vi "FPGA (Test Encoders).vi"() -> ()   [LabVIEW 2017]
uses:
  <vilib>/Platform/TimedLoop/XDataNode/timing_clust.ctl
  <vilib>/Platform/TimedLoop/XDataNode/nitl_modes.ctl
  <vilib>/Platform/TimedLoop/XDataNode/wakeup.ctl
  <vilib>/rvi/Emulation/niFpgaSctlEmulationGetInTimedLoop.vi
  <vilib>/rvi/Emulation/niFpgaEmulationReportErrorSimple.vi
  <vilib>/rvi/Emulation/niFpgaGetClockAttributes.vi
  <vilib>/rvi/Emulation/niFpgaCriticalErrorInLSC.vi
  <vilib>/rvi/Emulation/niFpgaEmulationIsFPGAContextNoSignature.vi
  <vilib>/rvi/DataTransferAndStorage/Container/Common/niFpgaContainerGetUniqueNameForEmu.vi
  <vilib>/rvi/Memory/Memory_Emulation/niFpgaMemoryEmulationCacheClearOnFirstRun.vi
  <vilib>/rvi/Memory/Memory_Emulation/nirvimemoryEmulationManagerCache_MakeExclusive.vi
  <vilib>/rvi/Memory/Memory_Emulation/niFpgaMemoryEmulationValidateCache.vi
  <vilib>/rvi/Memory/Memory_Emulation/nirvimemoryEmulationManagerCache_InsertValue.vi
  <vilib>/Utility/error.llb/Clear Errors.vi
  <vilib>/rvi/Memory/Memory_Emulation/nirvimemoryEmulationManagerCache_ReleaseExclusive.vi
  <vilib>/rvi/Memory/Memory_Emulation/nirvimemoryEmulationManagerCache_GetValue.vi
  <vilib>/rvi/Memory/Memory_Emulation/nirvimemoryEmulationManagerCache_SetValue.vi
  <vilib>/rvi/Emulation/niFpgaProcessEmulError.vi
  <vilib>/rvi/eio/common/nirviEmuTemplateMethod_errors.vi
  <vilib>/Platform/TimedLoop/XDataNode/XDataNode.xnode
  <vilib>/rvi/DataTransferAndStorage/Container/XNode/niFpgaContainer.xnode
  <vilib>/rvi/DataTransferAndStorage/Register/Emulation/niFpgaRegisterEmulation.vi
  <vilib>/eio/EIONode/EIONode.xnode
  <vilib>/Platform/TimedLoop/XDataNode/XDNodeRunTimeDep.lvlib
panel:
  out "dENC2_POS":fxp<+/-,54,31>
  out "dENC1_POS":fxp<+/-,54,31>
  out "ENC_2_loop_count":i32
  out "ENC_1_loop_count":i32
  out "ENC2_ticks":i32
  out "ENC1_ticks":i32
  out "ENC2_POS":fxp<+/-,64,27>
  out "ENC1_POS":fxp<+/-,64,29>
  in  "ENC2_DEBOUNCE_CYCLES":u16=5
  in  "LINK2_ENC_CNTS 2":i32
  in  "LINK2_UPDATE_ENC 2":bool
  out "Link 2 Counts 2":i32
  out "Link 1 Counts":i32
  in  "ENC_DEBOUNCE_CYCLES":u16=5
  in  "LINK1_ENC_CNTS":i32
  in  "LINK1_UPDATE_ENC":bool
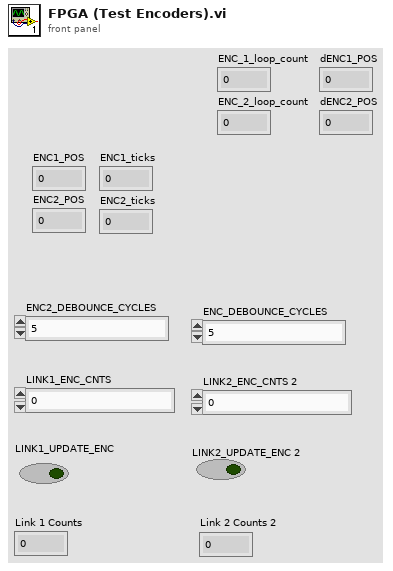
[diagram p1: front panel]
types:
  T1 = typedef "XDNodeRunTimeDep.lvlib/timing_clust.ctl" = cluster{"Expected End [f-1]":u64, "Actual End [f-1]":u64, "Finished Late? [f-1]":bool, "Expected End [i-1]":u64, "Actual End [i-1]":u64, "Finished Late? [i-1]":bool, "Expected Start [i]":u64, "Actual Start [i]":u64, "Expected Start [f]":u64, "Actual Start [f]":u64, "Source Name":string, "Structure Name":string, "Period":i64, "Deadline":i64, "Offset":i64, "Start":i64, "Priority":i32, "Timeout":i32, "Mode":T2, "Wakeup Reason":T3, "Error":errorcluster, "Source Type":string, "Secondary Source Type":string, "Global End Time":u64, "Global Start Time":u64, "Frame Duration":u64, "Iteration Duration":u64, "Assigned CPU":i32, "I/O Scan Engine Mode":u32}
  T2 = typedef "XDNodeRunTimeDep.lvlib/nitl_modes.ctl" = enum32{"No Change", "Process missed periods, maintain original phase", "Discard missed periods, maintain original phase", "Process missed periods, ignore original phase", "Discard missed periods, ignore original phase"}
  T3 = typedef "XDNodeRunTimeDep.lvlib/wakeup.ctl" = enum32{"Normal", "Aborted", "Asynchronous wakeup", "Timing source error", "Timed loop error", "Timeout"}
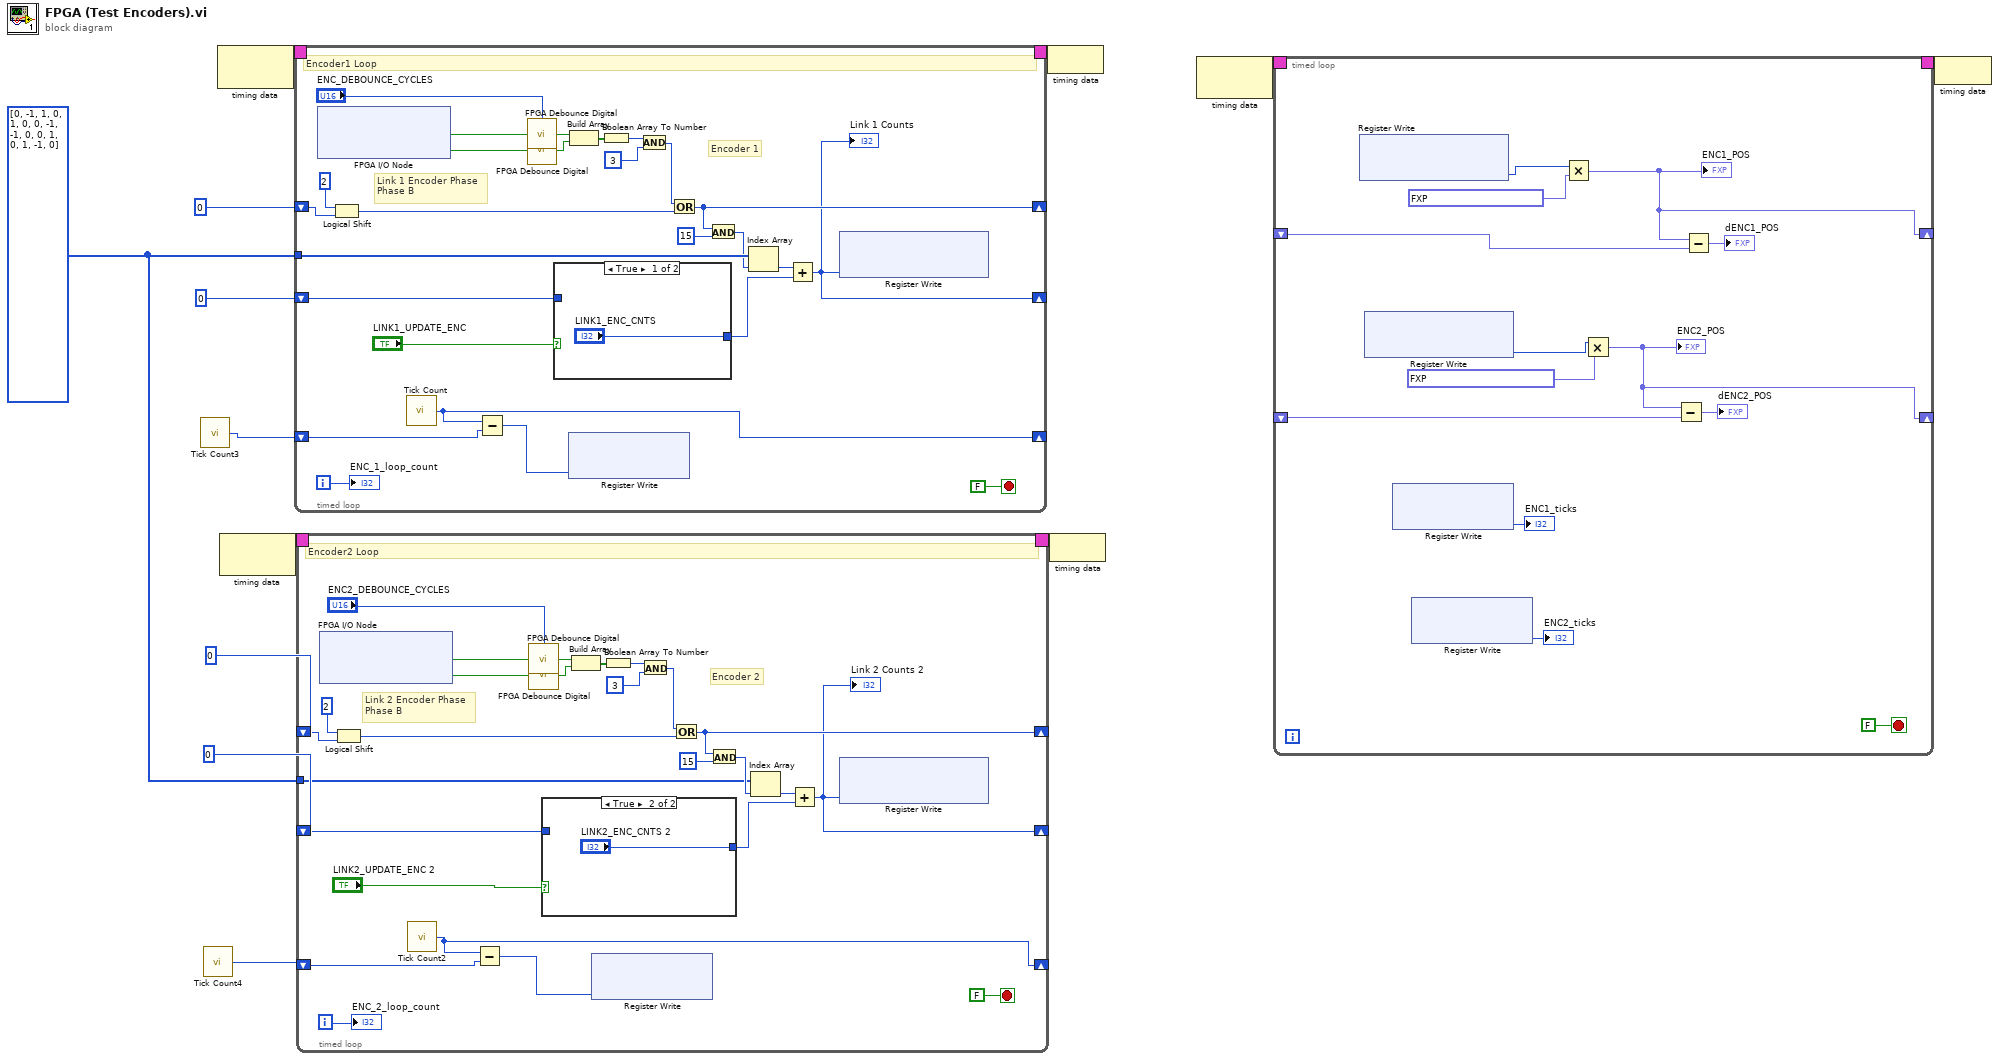
[diagram p0: block diagram]
diagram:
  w5 = i8[] [0, -1, 1, 0, 1, 0, 0, -1, -1, 0, 0, 1, 0, 1, -1, 0]
  n1 = call "Tick Count3"() -> ("Tick Count(Ticks)"=w2:u32)
  n2 = call "Tick Count4"() -> ("Tick Count(Ticks)"=w1:u32)
  n3 = node-c288() -> (w13:T1)  [unwired: 1 in]
  n4 = node-c288() -> (w9:T1)  [unwired: 1 in]
  n5 = timed-loop {
    timing: w13 -> [_]
    timing-out: [_] -> w12
    tunnel: w5 -> [w36]
    shift-right: [w29] -> _
    shift-left: u8 0 -> [w38]
    shift-right: [w18] -> _
    shift-left: 0 -> [w21]
    shift-right: [w16] -> _
    shift-left: w2 -> [w17]
    i -> [w14]
    stop <- FALSE stop-if-true
    # "Link 1 Encoder Phase \nPhase B"
    # "Encoder 1"
    # "Encoder1 Loop"
    n6 = xnode "FPGA I/O Node"() -> ("ConnectorC/DIO1"=w27:bool, "ConnectorC/DIO2"=w26:bool)  [unwired: 2 in, 2 out]
    n7 = Logical Shift(y=i16 2, x=w38) -> (x << y=w31:u8)
    n8 = call "Tick Count"() -> ("Tick Count(Ticks)"=w16:u32)
    n9 = Subtract(x=w16, y=w17) -> (x-y=w15:u32)
    n10 = call "FPGA Debounce Digital.vi"("Input Signal"=w27, "Cycles to Filter"="ENC_DEBOUNCE_CYCLES") -> ("Output Filtered Signal"=w25:bool)
    n11 = call "FPGA Debounce Digital.vi"("Input Signal"=w26, "Cycles to Filter"="ENC_DEBOUNCE_CYCLES") -> ("Output Filtered Signal"=w24:bool)
    n12 = case shown="True" "LINK1_UPDATE_ENC" {
      tunnel: w21 -> [_ w41]
      tunnel: ["LINK1_ENC_CNTS" w41] -> w20
      frame True {
      }
      frame False {
      }
    }
    n13 = xnode ("Register Write")("Data"=w15) -> ()  [unwired: 1 in, 1 out]
    n14 = Build Array(w25, w24) -> (w23:bool[])
    n15 = Boolean Array To Number(Boolean array=w23) -> (number=w34:u8)
    n16 = And(x=w34, y=u8 3) -> (x .and. y?=w32:u8)
    n17 = Or(x=w32, y=w31) -> (x .or. y?=w29:u8)
    n18 = And(x=w29, y=u8 15) -> (x .and. y?=w30:u8)
    n19 = Index Array(array=w36, index=w30) -> (element=w28:i8)
    n20 = Add(x=w28, y=w20) -> (x+y=w18:i32)
    "Link 1 Counts" <- w18
    n21 = xnode ("Register Write")("Data"=w18) -> ()  [unwired: 1 in, 1 out]
    "ENC_1_loop_count" <- w14
  }
  n22 = timed-loop {
    timing: w9 -> [_]
    timing-out: [_] -> w8
    tunnel: w5 -> [w54]
    shift-right: [w52] -> _
    shift-left: u8 0 -> [w53]
    shift-right: [w51] -> _
    shift-left: 0 -> [w49]
    shift-right: [w46] -> _
    shift-left: w1 -> [w47]
    i -> [w44]
    stop <- FALSE stop-if-true
    # "Link 2 Encoder Phase \nPhase B"
    # "Encoder 2"
    # "Encoder2 Loop"
    n23 = xnode "FPGA I/O Node"() -> ("ConnectorC/DIO5"=w60:bool, "ConnectorC/DIO6"=w59:bool)  [unwired: 2 in, 2 out]
    n24 = Logical Shift(y=i16 2, x=w53) -> (x << y=w63:u8)
    n25 = call "Tick Count2"() -> ("Tick Count(Ticks)"=w46:u32)
    n26 = Subtract(x=w46, y=w47) -> (x-y=w45:u32)
    n27 = call "FPGA Debounce Digital.vi"("Input Signal"=w60, "Cycles to Filter"="ENC2_DEBOUNCE_CYCLES") -> ("Output Filtered Signal"=w58:bool)
    n28 = call "FPGA Debounce Digital.vi"("Input Signal"=w59, "Cycles to Filter"="ENC2_DEBOUNCE_CYCLES") -> ("Output Filtered Signal"=w57:bool)
    n29 = case shown="True" "LINK2_UPDATE_ENC 2" {
      tunnel: w49 -> [w70 _]
      tunnel: [w70 "LINK2_ENC_CNTS 2"] -> w55
      frame False {
      }
      frame True {
      }
    }
    n30 = Build Array(w58, w57) -> (w56:bool[])
    n31 = xnode ("Register Write")("Data"=w45) -> ()  [unwired: 1 in, 1 out]
    n32 = Boolean Array To Number(Boolean array=w56) -> (number=w66:u8)
    n33 = And(x=w66, y=u8 3) -> (x .and. y?=w64:u8)
    n34 = Or(x=w64, y=w63) -> (x .or. y?=w52:u8)
    n35 = And(x=w52, y=u8 15) -> (x .and. y?=w62:u8)
    n36 = Index Array(array=w54, index=w62) -> (element=w61:i8)
    n37 = Add(x=w61, y=w55) -> (x+y=w51:i32)
    "Link 2 Counts 2" <- w51
    n38 = xnode ("Register Write")("Data"=w51) -> ()  [unwired: 1 in, 1 out]
    "ENC_2_loop_count" <- w44
  }
  n39 = node-c288(w12) -> ()
  n40 = node-c288(w8) -> ()
  n41 = node-c288() -> (w4:T1)  [unwired: 1 in]
  n42 = timed-loop {
    timing: w4 -> [_]
    timing-out: [_] -> w3
    shift-right: [w78] -> _
    shift-left: _ -> [w79]
    shift-right: [w75] -> _
    shift-left: _ -> [w76]
    stop <- FALSE stop-if-true
    n43 = xnode ("Register Write")() -> ("Data"=w85:i32)  [unwired: 1 in, 1 out]
    n44 = xnode ("Register Write")() -> ("Data"=w83:i32)  [unwired: 1 in, 1 out]
    n45 = xnode ("Register Write")() -> ("Data"=→"ENC1_ticks":i32)  [unwired: 1 in, 1 out]
    n46 = xnode ("Register Write")() -> ("Data"=→"ENC2_ticks":i32)  [unwired: 1 in, 1 out]
    n47 = Multiply(x=w85, y=fxp<+,21,-2> 0.2197270393371582) -> (x*y=w78:fxp<+/-,53,30>)
    "ENC1_POS" <- w78
    n48 = Multiply(x=w83, y=fxp<+,21,-2> 0.1255580186843872) -> (x*y=w75:fxp<+/-,53,30>)
    "ENC2_POS" <- w75
    n49 = Subtract(x=w75, y=w76) -> (x-y=→"dENC2_POS":fxp<+/-,54,31>)
    n50 = Subtract(x=w78, y=w79) -> (x-y=→"dENC1_POS":fxp<+/-,54,31>)
  }
  n51 = node-c288(w3) -> ()
